vi "RAM Test.vi"(11 "RAMFail":bool) -> (0 "error out":errorcluster, 3 "Result":bool)   [LabVIEW 2013]
doc: "Tests the Random Access Memory (RAM)."
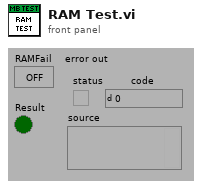
[diagram p1: front panel]
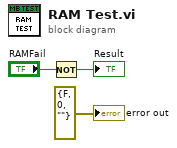
[diagram p0: block diagram]
diagram:
  n1 = Not(x="RAMFail") -> (.not. x?=→"Result":bool)
  "error out" <- errorcluster {"status"=FALSE, "code"=0, "source"=""} ("error out")
